vi "Pre Launch Init.vi"(11 "Master Controller in":refnum<class "EMS User Interface.lvclass">) -> (0 "error out":errorcluster, 3 "Master Controller out":refnum<class "EMS User Interface.lvclass">)   [LabVIEW 2018, in "EMS User Interface Actor.lvlib" / "EMS User Interface.lvclass"]
doc: "(<B>Filename</B>: Actor Framework.lvlib:Actor.lvclass:Pre Launch Init.vi)\n\nDefines behavior that occurs after the Launch Nested Actor method is invoked but before the actor's Actor Core method begins running.\n\nBy default, this method does nothing. A descendant class may override it to define behavior."
uses:
  EMS User Interface.lvclass
  C:/Users/Administrator/Desktop/LabVIEW EMS/EMS Generic Actor/EMS Generic/EMS Generic.lvclass
  EMS Generic Actor/EMS Generic/Controls/Device Information Cluster.ctl
  EMS Generic Actor/EMS Generic/Controls/Device State.ctl
  <vilib>/ORNL/CSEISMIC DDS/CSEISMIC DDS Base/Data Types/IED_Status.ctl
  <vilib>/ORNL/CSEISMIC DDS/CSEISMIC DDS Base/Data Types/Controls/DeviceID.ctl
  <vilib>/ORNL/CSEISMIC DDS/CSEISMIC DDS Base/Data Types/Controls/Timestamp.ctl
  EMS Generic Actor/EMS Generic/Controls/Global Configuration.ctl
  EMS Generic Actor/EMS Generic/EMS Generic.lvclass/EMS Generic.ctl
  EMS Core/EMS/Controls/Microgrid State.ctl
  Controls/Master Controller User Events.ctl
  EMS User Interface.lvclass/EMS User Interface.ctl
  EMS Generic Actor/EMS Generic/EMS Generic.lvclass
  EMS Core/EMS/EMS.lvclass
  <vilib>/ORNL/CSEISMIC DDS/CSEISMIC DDS Base/CSEISMIC DDS.lvclass
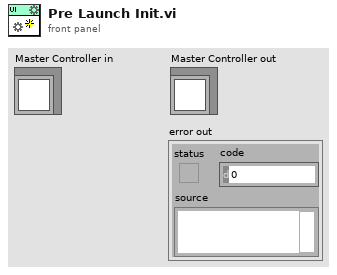
[diagram p1: front panel]
types:
  T1 = typedef "EMS Generic Actor.lvlib/EMS Generic.lvclass/Device Information Cluster.ctl" = cluster{"Device State":T2, "data":variant}
  T2 = typedef "EMS Generic Actor.lvlib/EMS Generic.lvclass/Device State.ctl" = enum16{"Invalid", "Clear", "DevIDs in Config", "DevIDs on uGrid", "DevIDs not on uGrid", "Update IED_Status", "Update DER_Status", "Update DER_Measurement", "Update SmartRelay_Measurement"}
  T3 = typedef "CSEISMIC DDS.lvlib/CSEISMIC DDS.lvclass/IED_Status.ctl" = cluster{"DeviceID":T4, "Timestamp":T5, "MicrogridID":u8, "Active":bool, "Inactive":bool, "Error":i32, "Fault":bool, "ErrorString":string}
  T4 = typedef "CSEISMIC DDS.lvlib/CSEISMIC DDS.lvclass/DeviceID.ctl" = string
  T5 = typedef "CSEISMIC DDS.lvlib/CSEISMIC DDS.lvclass/Timestamp.ctl" = cluster{"Seconds":u64, "Remainder":u64}
  T6 = typedef "EMS Generic Actor.lvlib/EMS Generic.lvclass/Global Configuration.ctl" = cluster{"Microgrid ID":u8, "VF Device ID":T4, "Ongrid VF Priority":T4[], "Offgrid VF Priority":T4[], "AutoSwap Offgrid VF":u32, "AutoSwap Offgrid VF Delay (sec)":dbl, "AutoSwap Resynch VF":u32, "PCC Device ID":T4, "Device ID Array":T4[], "Nominal Voltage":dbl, "Nominal Frequency":dbl, "Resynch Timeout (sec)":dbl, "Island VF Activate Timeout (sec)":dbl, "Island PCC Target Power (kW)":dbl, "Island PCC Target Power Timeout (sec)":dbl, "Island Grid Settle Time (sec)":dbl, "Island PCC Failure Timeout (sec)":dbl, "Activation Devices Present Timeout (sec)":dbl, "Activation Devices Activated Timeout (sec)":dbl, "Blackstart VF GenMode Wait (sec)":dbl, "Blackstart VF DERCtrl Wait (sec)":dbl, "Blackstart Success Wait (sec)":dbl, "OnGrid Optimization Delay (sec)":dbl, "OffGrid Optimization Delay (sec)":dbl, "Resynch Frequency (Hz)":dbl, "Optimization Path":string}
  T7 = typedef "EMS Core.lvlib/EMS.lvclass/Microgrid State.ctl" = enum16{"Discovery", "Commissioning", "Activation", "Blackstart", "OnGrid", "OffGrid", "Island", "Resynchronization", "Manual", "Shutdown", "Stop"}
  T8 = typedef "EMS User Interface Actor.lvlib/EMS User Interface.lvclass/Master Controller User Events.ctl" = cluster{"Current State":refnum<user-event>, "Current Status":refnum<user-event>, "Device List":refnum<user-event>, "P Meas":refnum<user-event>, "Q Meas":refnum<user-event>, "P Set Max":refnum<user-event>, "Q Set Max":refnum<user-event>, "IED_Status":refnum<user-event>, "Device State Information":refnum<user-event>}
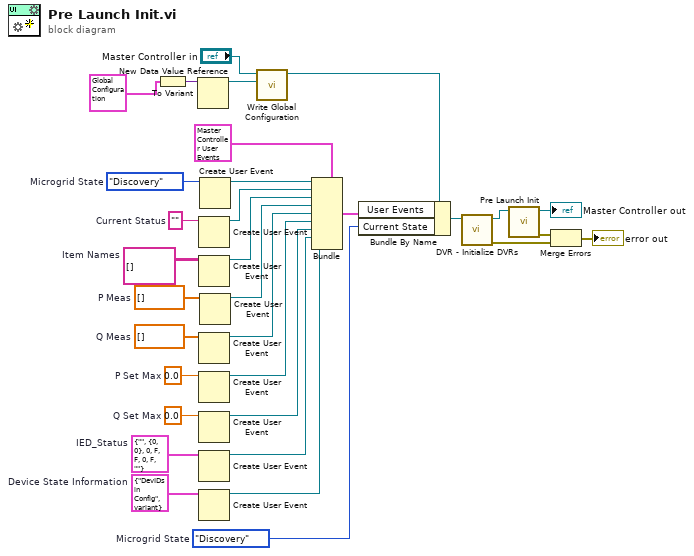
[diagram p0: block diagram]
diagram:
  w2 = T1 {"Device State"=enum."DevIDs in Config", "data"=variant}  # Device State Information
  w3 = T3 {"DeviceID"="", "Timestamp"={"Seconds"=0, "Remainder"=0}, "MicrogridID"=0, "Active"=FALSE, "Inactive"=FALSE, "Error"=0, "Fault"=FALSE, "ErrorString"=""}  # IED_Status
  w8 = 0.0  # Q Set Max
  w9 = 0.0  # P Set Max
  w12 = dbl[] []  # Q Meas
  w14 = dbl[] []  # P Meas
  w16 = string[][] []  # Item Names
  w24 = Microgrid_State."Discovery"  # Microgrid State
  w25 = Microgrid_State."Discovery"  # Microgrid State
  w30 = ""  # Current Status
  n1 = To Variant(anything=T6 {"Microgrid ID"=1, "VF Device ID"="", "Ongrid VF Priority"=[], "Offgrid VF Priority"=[], "AutoSwap Offgrid VF"=0, "AutoSwap Offgrid VF Delay (sec)"=0.0, "AutoSwap Resynch VF"=0, "PCC Device ID"="", "Device ID Array"=[], "Nominal Voltage"=0.0, "Nominal Frequency"=0.0, "Resynch Timeout (sec)"=0.0, "Island VF Activate Timeout (sec)"=0.0, "Island PCC Target Power (kW)"=0.0, "Island PCC Target Power Timeout (sec)"=0.0, "Island Grid Settle Time (sec)"=0.0, "Island PCC Failure Timeout (sec)"=0.0, "Activation Devices Present Timeout (sec)"=0.0, "Activation Devices Activated Timeout (sec)"=0.0, "Blackstart VF GenMode Wait (sec)"=0.0, "Blackstart VF DERCtrl Wait (sec)"=0.0, "Blackstart Success Wait (sec)"=0.0, "OnGrid Optimization Delay (sec)"=0.0, "OffGrid Optimization Delay (sec)"=0.0, "Resynch Frequency (Hz)"=0.0, "Optimization Path"=""} ("Global Configuration")) -> (Variant=w4:variant)
  n2 = New Data Value Reference(data value=w4) -> (data value reference=w21:refnum<data-value>)  [unwired: 1 in, 1 out]
  n3 = Create User Event(user event datatype=w30) -> (user event=w28:refnum<user-event>)  [unwired: 1 in, 1 out]
  n4 = Create User Event(user event datatype=w16) -> (user event=w15:refnum<user-event>)  [unwired: 1 in, 1 out]
  n5 = Create User Event(user event datatype=w12) -> (user event=w11:refnum<user-event>)  [unwired: 1 in, 1 out]
  n6 = Create User Event(user event datatype=w9) -> (user event=w10:refnum<user-event>)  [unwired: 1 in, 1 out]
  n7 = Create User Event(user event datatype=w8) -> (user event=w7:refnum<user-event>)  [unwired: 1 in, 1 out]
  n8 = Create User Event(user event datatype=w3) -> (user event=w6:refnum<user-event>)  [unwired: 1 in, 1 out]
  n9 = Create User Event(user event datatype=w2) -> (user event=w1:refnum<user-event>)  [unwired: 1 in, 1 out]
  n10 = Create User Event(user event datatype=w24) -> (user event=w29:refnum<user-event>)  [unwired: 1 in, 1 out]
  n11 = Create User Event(user event datatype=w14) -> (user event=w13:refnum<user-event>)  [unwired: 1 in, 1 out]
  n12 = call "Write Global Configuration.vi"("Global Configuration"=w21, "EMS Generic in"="Master Controller in") -> ("EMS Generic out"=w22:refnum<class "EMS User Interface.lvclass">)  [unwired: 9 in]
  n13 = Bundle(cluster=T8 {"Current State"=refnum, "Current Status"=refnum, "Device List"=refnum, "P Meas"=refnum, "Q Meas"=refnum, "P Set Max"=refnum, "Q Set Max"=refnum, "IED_Status"=refnum, "Device State Information"=refnum} ("User Events"), "Current State"=w29, "Current Status"=w28, "Device List"=w15, "P Meas"=w13, "Q Meas"=w11, "P Set Max"=w10, "Q Set Max"=w7, "IED_Status"=w6, "Device State Information"=w1) -> (w27:T8)
  n14 = Bundle By Name(cluster=w22, "User Events"=w27, "Current State"=w25) -> (w20:refnum<class "EMS User Interface.lvclass">)
  n15 = call "DVR - Initialize DVRs.vi"("EMS Generic in"=w20) -> ("error out"=w17:errorcluster, "EMS Generic out"=w19:refnum<class "EMS User Interface.lvclass">)  [unwired: 9 in]
  n16 = call-parent "Pre Launch Init.vi"("EMS Generic in"=w19) -> ("error out"=w32:errorcluster, "EMS Generic out"=→"Master Controller out":refnum<class "EMS User Interface.lvclass">)  [unwired: 9 in]
  n17 = Merge Errors(w32, w17) -> (→"error out":errorcluster)
